vi "Normal Drive.vi"(0 "Joy X":dbl, 1 "Joy Y":dbl, 2 "Short Radius (Inches)":dbl, 3 "Long Radius (Inches)":dbl, 5 "Robot Orientation":T1) -> (6 "Front Left Angle Out":dbl, 7 "Front Right Angle Out":dbl, 8 "Left Speed Out":dbl, 9 "Right Speed Out":dbl)   [LabVIEW 2012]
uses:
  Controls/Robot Orientation.ctl
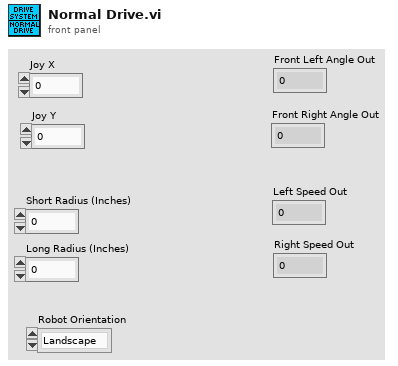
[diagram p1: front panel]
types:
  T1 = typedef "Robot Orientation.ctl" = enum16{"Landscape", "Portrait"}
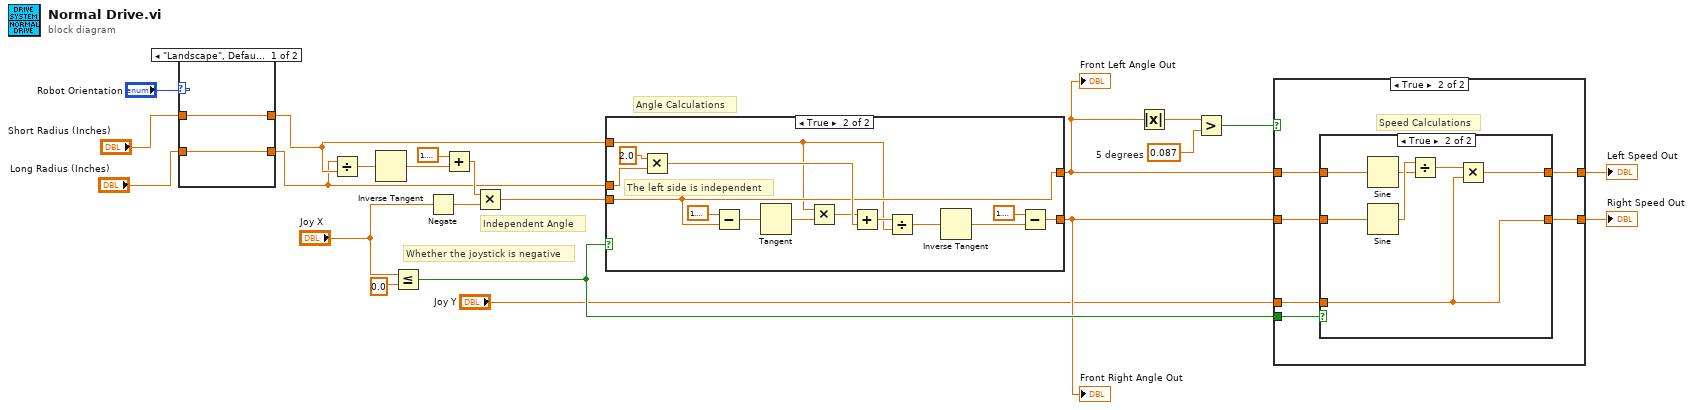
[diagram p0: block diagram]
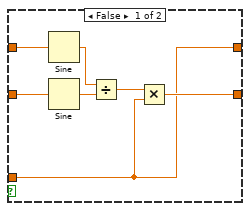
[diagram p4: hidden frame]
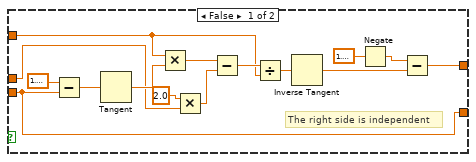
[diagram p5: hidden frame]
diagram:
  w7 = 0.087  # 5 degrees
  # "Angle Calculations"
  # "Whether the joystick is negative"
  # "Independent Angle"
  n1 = case shown="\"Landscape\", Default" "Robot Orientation" {
    tunnel: "Short Radius (Inches)" -> [w24 w26]
    tunnel: "Long Radius (Inches)" -> [w23 w25]
    tunnel: [w24 w25] -> w3
    tunnel: [w23 w26] -> w1
    frame "Landscape", Default {
    }
    frame "Portrait" {
    }
  }
  n2 = Divide(x=w1, y=w3) -> (x/y=w21:dbl)
  n3 = Inverse Tangent(1:w21) -> (0:w20:dbl)
  n4 = Less Or Equal?(x="Joy X", y=0.0) -> (x <= y?=w15:bool)
  n5 = Negate(x="Joy X") -> (-x=w18:dbl)
  n6 = Add(x=1.5707963267948966, y=w20) -> (x+y=w19:dbl)
  n7 = Multiply(x=w19, y=w18) -> (x*y=w16:dbl)
  n8 = case shown="True" w15 {
    tunnel: w16 -> [w28 w47]
    tunnel: [w27 w47] -> w9
    tunnel: [w28 w46] -> w14
    tunnel: w3 -> [w30 w44]
    tunnel: w1 -> [w29 w45]
    frame False {
      # "The right side is independent"
      n9 = Subtract(x=1.5707963267948966, y=w28) -> (x-y=w33:dbl)
      n10 = Tangent(1:w33) -> (0:w34:dbl)
      n11 = Multiply(x=w30, y=w34) -> (x*y=w41:dbl)
      n12 = Multiply(x=2.0, y=w29) -> (x*y=w35:dbl)
      n13 = Subtract(x=w41, y=w35) -> (x-y=w37:dbl)
      n14 = Divide(x=w37, y=w30) -> (x/y=w38:dbl)
      n15 = Inverse Tangent(1:w38) -> (0:w31:dbl)
      n16 = Negate(x=1.5707963267948966) -> (-x=w39:dbl)
      n17 = Subtract(x=w39, y=w31) -> (x-y=w27:dbl)
    }
    frame True {
      # "The left side is independent"
      n18 = Multiply(x=2.0, y=w45) -> (x*y=w51:dbl)
      n19 = Subtract(x=1.5707963267948966, y=w47) -> (x-y=w53:dbl)
      n20 = Tangent(1:w53) -> (0:w52:dbl)
      n21 = Multiply(x=w44, y=w52) -> (x*y=w43:dbl)
      n22 = Add(x=w43, y=w51) -> (x+y=w49:dbl)
      n23 = Divide(x=w49, y=w44) -> (x/y=w48:dbl)
      n24 = Inverse Tangent(1:w48) -> (0:w55:dbl)
      n25 = Subtract(x=1.5707963267948966, y=w55) -> (x-y=w46:dbl)
    }
  }
  "Front Left Angle Out" <- w9
  "Front Right Angle Out" <- w14
  n26 = Absolute Value(x=w9) -> (abs(x)=w8:dbl)
  n27 = Greater?(x=w8, y=w7) -> (0:w6:bool)
  n28 = case shown="True" w6 {
    tunnel: w15 -> [_ w62]
    tunnel: w14 -> [_ w61]
    tunnel: w9 -> [_ w60]
    tunnel: [w56 w59] -> w13
    tunnel: [w56 w58] -> w12
    tunnel: "Joy Y" -> [w56 w57]
    frame False {
    }
    frame True {
      # "Speed Calculations"
      n29 = case shown="True" w62 {
        tunnel: w61 -> [w65 w75]
        tunnel: w60 -> [w66 w76]
        tunnel: [w64 w70] -> w59
        tunnel: [w63 w73] -> w58
        tunnel: w57 -> [w63 w70]
        frame False {
          n30 = Sine(x=w66) -> (sin(x)=w67:dbl)
          n31 = Sine(x=w65) -> (sin(x)=w68:dbl)
          n32 = Divide(x=w67, y=w68) -> (x/y=w69:dbl)
          n33 = Multiply(x=w69, y=w63) -> (x*y=w64:dbl)
        }
        frame True {
          n34 = Sine(x=w76) -> (sin(x)=w71:dbl)
          n35 = Sine(x=w75) -> (sin(x)=w72:dbl)
          n36 = Divide(x=w72, y=w71) -> (x/y=w74:dbl)
          n37 = Multiply(x=w74, y=w70) -> (x*y=w73:dbl)
        }
      }
    }
  }
  "Right Speed Out" <- w13
  "Left Speed Out" <- w12
